vi "CH_LM Measurement Fetch Data.vi"(0 "Meter Index":i32, 3 "All Records? (F)":bool, 5 "error in (no error)":errorcluster, 7 "Timeout / ms (1000)":i32=1000) -> (14 "Meter Index":i32, 16 "Data OK":bool, 17 "Data Array":T1[](array[typedef]) {"Flags" format="%.0b"; "Unit ID" format="%.0b"; "Quad Distance"."Y" format="%#.1f"; "Quad Distance"."X" format="%#.1f"; "Value" format="%#.7e"}, 18 "timed out?":bool, 19 "error out":errorcluster)   [LabVIEW 2017, in "CH_LM.lvlib"]
doc: "This VI reads the streaming data and converts it to LabVIEW datatypes. \nIf the LabMax streaming mode is enabled the streaming data is send with approximatly 10 Hz.\n\n- In case of USB communication mode this VI waits for Streaming Packets.\n- In case of GPIB and RS232 communication mode this VI waits for Service Request (SRQ) and fetches all available data records.\n\n<B>Attention:</B> This VI is intentionally reentrant!\n\n<B>Note:</B> Data without Header is not supported in this revision.\n\nThe meter will internally generate a data record according to the following rules:\n- With every pulse when a pyroelectric probe is attached and if Joules mode is selected\n- Every 300 ms when a pyroelectric probe is attached and if Watts mode is selected\n- With every pulse when a thermopile probe is attached and if Joules mode is selected \n- When a measurement sample is taken when a thermopile or optical probe is attached and if Watts mode is selected\n\nSince thermopile and optical power measurements are continuous in nature (not event based as with pyroelectric probes), the delivery of this data may be configured as a stream of sampled points or simply the last point recorded. Refer to CH_LM Config Measurement Delivery Mode.vi."
uses:
  CH_LM.lvlib
  CH_LM Streaming Data.ctl
  _CH_LM/CH_LM Action Enumeration.ctl
  _CH_LM/CH_LM Event Cluster.ctl
  CH_LM_App/CH_LM Globals Debug-Status.vi
  CH_LM App.lvlib
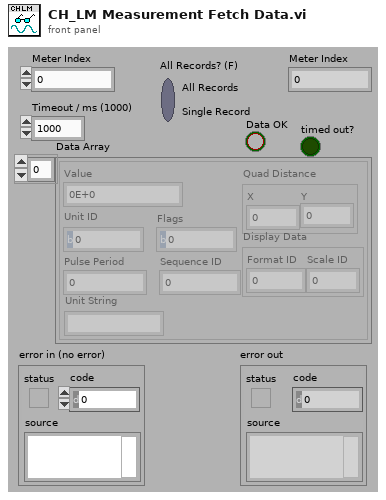
[diagram p1: front panel]
types:
  T1 = typedef "CH_LM.lvlib/CH_LM Streaming Data.ctl" = cluster{"Value":sgl, "Quad Distance":cluster{"X":sgl, "Y":sgl}, "Display Data":cluster{"Format ID":u8, "Scale ID":u8}, "Unit ID":u8, "Flags":u32, "Pulse Period":u32, "Sequence ID":u32, "Unit String":string}
  T2 = typedef "CH_LM.lvlib/CH_LM Action Enumeration.ctl" = enum16{"add", "read", "read by serial", "set", "remove", "delete", "Clear Shift-Register", ""}
  T3 = typedef "CH_LM.lvlib/CH_LM Event Cluster.ctl" = cluster{"Event Name":string, "Meter Index":i32, "Serial  Number":string, "Data":string, "iStreamingPacket":variant}
  T4 = typedef "CH_LM.lvlib/CH_LM Communication Mode.ctl" = enum16{"None", "USB", "GPIB", "RS232"}
  T5 = typedef "CH_LM.lvlib/CH_LM Meter Info.ctl" = cluster{"Meter Index":i32, "Serial Number":string, "Queue Cluster":T6, "Data Header":bool, "Data Tokens":T7[]}
  T6 = typedef "CH_LM.lvlib/CH_LM Queue Cluster.ctl" = cluster{"Streaming Queue":refnum<queue>, "Asynch Notifier":refnum<notifier>}
  T7 = typedef "CH_LM.lvlib/CH_LM Data Token.ctl" = enum16{"Raw data", "Quad distance", "Formated data", "Unit", "Pulse period", "Flags", "Sequence ID"}
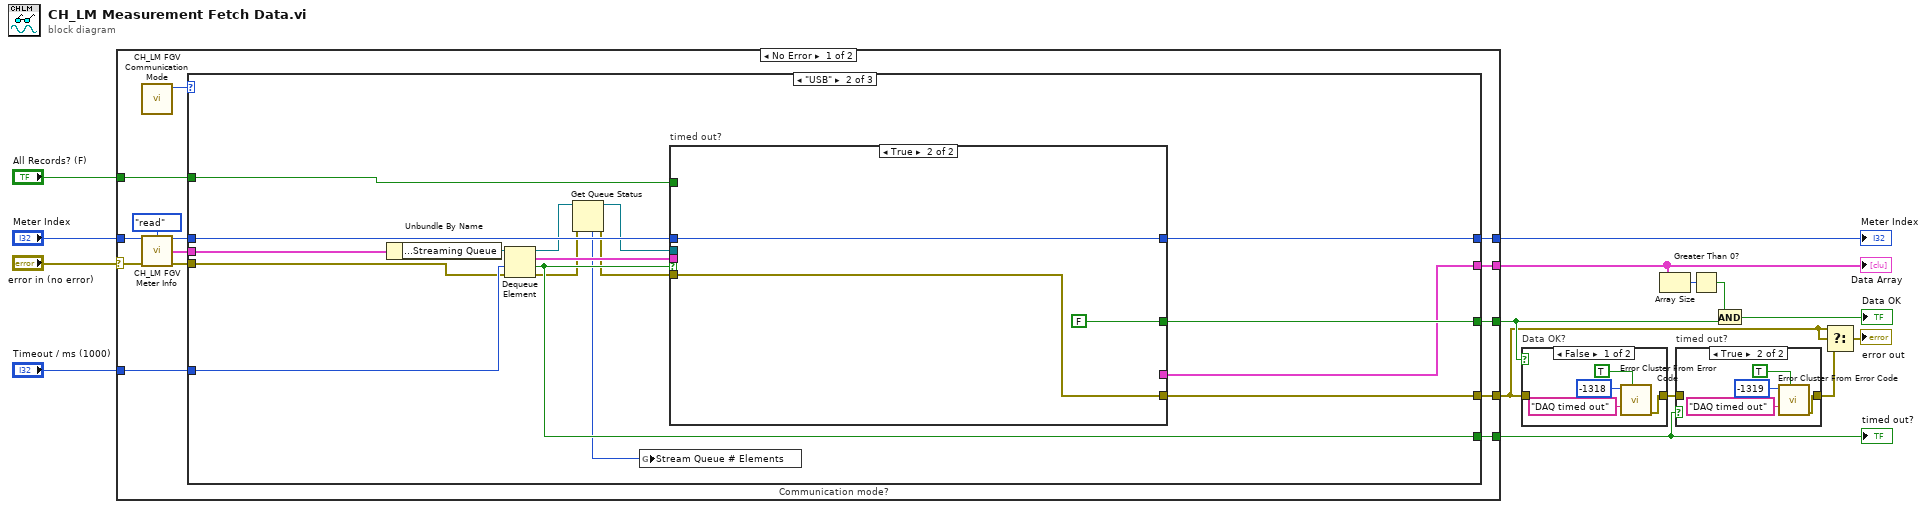
[diagram p0: block diagram]
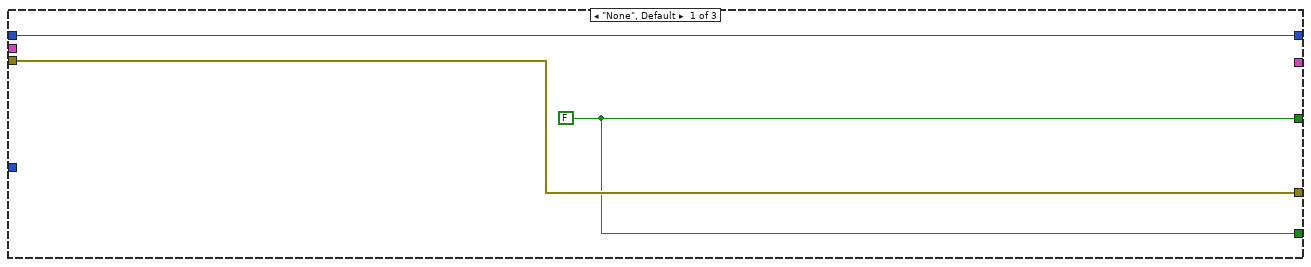
[diagram p4: hidden frame]
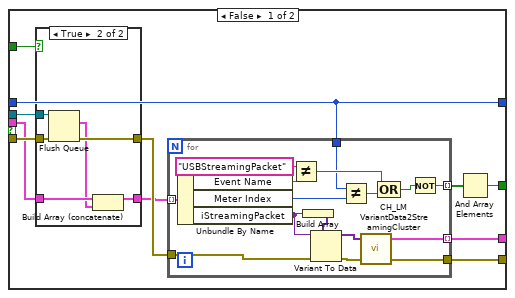
[diagram p5: hidden frame]
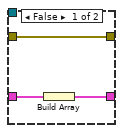
[diagram p6: hidden frame]
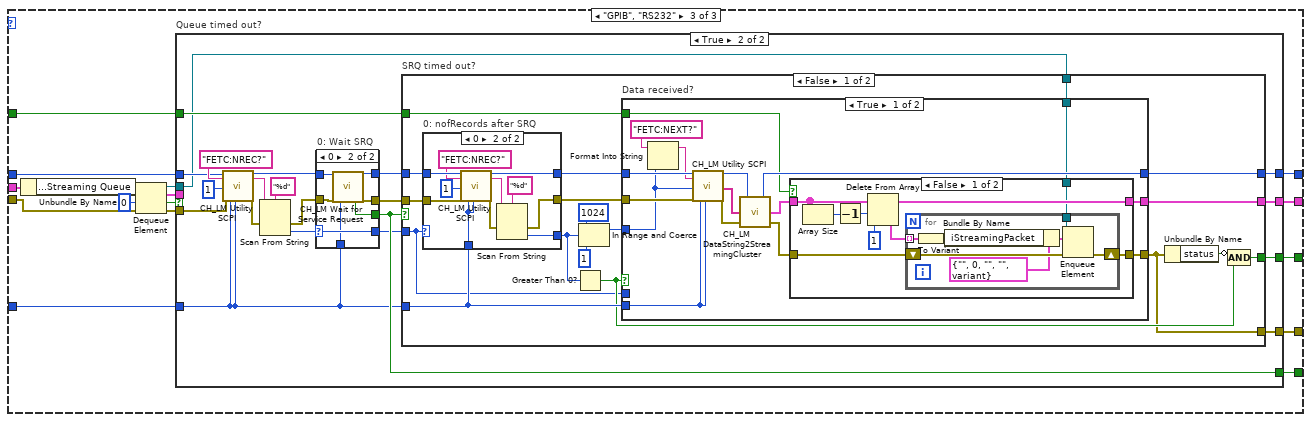
[diagram p7: hidden frame]
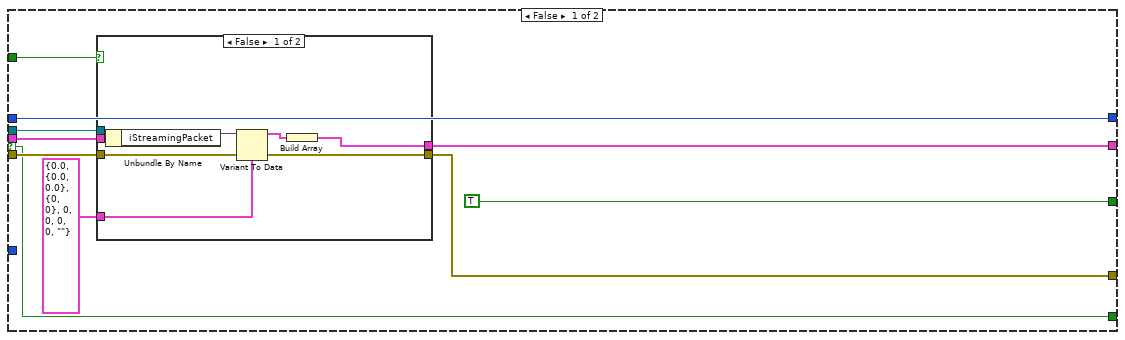
[diagram p8: hidden frame]
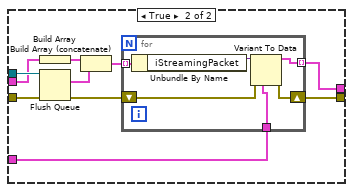
[diagram p9: hidden frame]
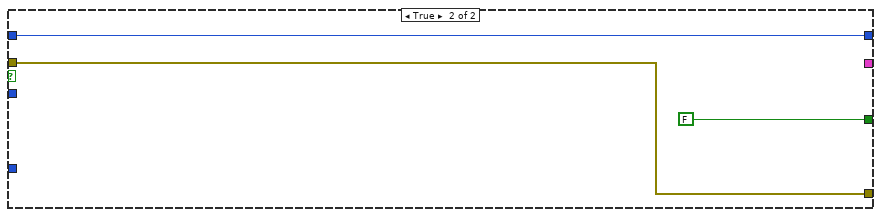
[diagram p14: hidden frame]
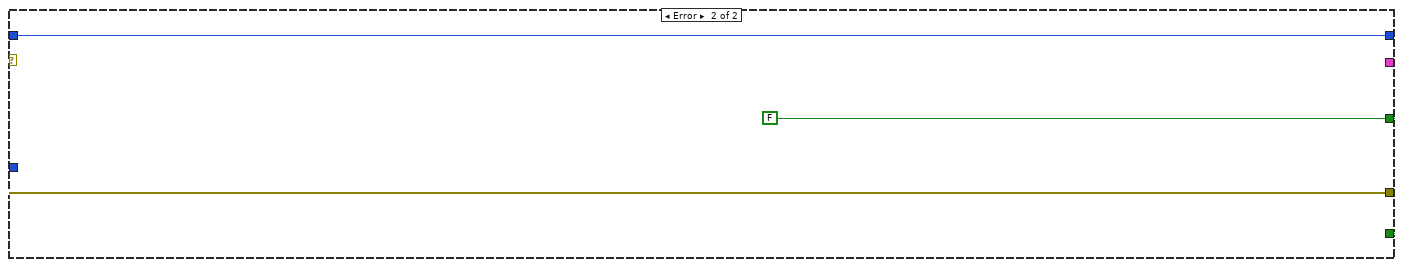
[diagram p15: hidden frame]
diagram:
  n1 = case shown="No Error" "error in (no error)" {
    selector: "error in (no error)" -> [w26 w242]
    tunnel: [w23 w242] -> w3
    tunnel: "Meter Index" -> [w25 w241]
    tunnel: [w19 w241] -> w13
    tunnel: [w22 _] -> w10
    tunnel: [w21 w240] -> w4
    tunnel: "Timeout / ms (1000)" -> [w20 _]
    tunnel: "All Records? (F)" -> [w17 _]
    tunnel: [w16 w240] -> w6
    frame No Error {
      n2 = call "CH_LM FGV Communication Mode.vi"() -> ("Communication Mode"=w18:T4)  [unwired: 3 in, 5 out]
      n3 = call "CH_LM FGV Meter Info.vi"("Meter Index"=w25, "Action (read)"=CH_LM_Action_Enumeration."read", "error in (no error)"=w26) -> ("Meter Index out"=w24:i32, "Meter Info"=w29:T5, "error out"=w28:errorcluster)  [unwired: 2 in, 8 out]
      n4 = case "Communication mode?" shown="\"USB\"" w18 {
        tunnel: w20 -> [_ w49 w97]
        tunnel: w29 -> [_ w48 w96]
        tunnel: w28 -> [w32 w46 w94]
        tunnel: w24 -> [w31 w44 w98]
        tunnel: [w32 w43 w102] -> w23
        tunnel: [_ w38 w103] -> w22
        tunnel: [w30 w45 w101] -> w21
        tunnel: [w31 w42 w104] -> w19
        tunnel: w17 -> [_ w40 w100]
        tunnel: [w30 w39 w99] -> w16
        frame "None", Default {
          w30 = FALSE
        }
        frame "USB" {
          n5 = Unbundle By Name(w48) -> ("Queue Cluster.Streaming Queue"=w47:refnum<queue>)
          n6 = Dequeue Element(queue=w47, timeout in ms (-1)=w49, error in (no error)=w46) -> (queue out=w37:refnum<queue>, element=w41:T3, timed out?=w39:bool, error out=w35:errorcluster)
          n7 = Get Queue Status(queue=w37, error in (no error)=w35) -> (queue out=w36:refnum<queue>, error out=w34:errorcluster, # elements in queue=w33:i32)  [unwired: 1 in, 5 out]
          n8 = global write "CH_LM Globals Debug-Status.vi" "Stream Queue # Elements"(w33) -> ()
          n9 = case "timed out?" shown="True" w39 {
            tunnel: [w59 w86] -> w43
            tunnel: w44 -> [w51 w88]
            tunnel: [w58 _] -> w38
            tunnel: [w57 FALSE] -> w45
            tunnel: w36 -> [w56 _]
            tunnel: w34 -> [w55 w86]
            tunnel: w41 -> [w53 _]
            tunnel: [w51 w88] -> w42
            tunnel: w40 -> [w50 _]
            frame False {
              n10 = case shown="True" w50 {
                tunnel: w56 -> [_ w69]
                tunnel: w55 -> [w63 w68]
                tunnel: [w63 w67] -> w54
                tunnel: w53 -> [w62 w66]
                tunnel: [w61 w64] -> w52
                frame False {
                  n11 = Build Array(w62) -> (w61:T3[])
                }
                frame True {
                  n12 = Flush Queue(queue=w69, error in (no error)=w68) -> (remaining elements=w65:T3[], error out=w67:errorcluster)  [unwired: 1 out]
                  n13 = Build Array (concatenate)(w66, w65) -> (w64:T3[])
                }
              }
              n14 = for {
                tunnel: [w80] -> w60 mode=indexing
                tunnel: [w72] -> w59
                tunnel: w51 -> [w73]
                tunnel: w54 -> [w76]
                tunnel: w52 -> [w75] mode=indexing
                tunnel: [w70] -> w58 mode=indexing
                n15 = Unbundle By Name(w75) -> ("Event Name"=w85:string, "Meter Index"=w77:i32, "iStreamingPacket"=w78:variant)
                n16 = Not Equal?(x="USBStreamingPacket", y=w85) -> (x != y?=w83:bool)
                n17 = Build Array(w78) -> (w79:variant[])
                n18 = Variant To Data(error in=w76, type=w79, Variant=w78) -> (data=w71:variant[], error out=w74:errorcluster)
                n19 = Not Equal?(x=w73, y=w77) -> (x != y?=w82:bool)
                n20 = call "CH_LM VariantData2StreamingCluster.vi"("error in (no error)"=w74, "Streaming Data"=w71) -> ("error out"=w72:errorcluster, "Streaming Data Cluster"=w70:T1)  [unwired: 1 in, 1 out]
                n21 = Compound Arithmetic op=OR(w83, w82) -> (w81:bool)
                n22 = Not(x=w81) -> (.not. x?=w80:bool)
              }
              n23 = And Array Elements(Boolean array=w60) -> (logical AND=w57:bool)
            }
            frame True {
            }
          }
        }
        frame "GPIB", "RS232" {
          n24 = Unbundle By Name(w96) -> ("Queue Cluster.Streaming Queue"=w95:refnum<queue>)
          n25 = Dequeue Element(queue=w95, timeout in ms (-1)=0, error in (no error)=w94) -> (queue out=w89:refnum<queue>, element=w90:T3, timed out?=w91:bool, error out=w93:errorcluster)
          n26 = case "Queue timed out?" shown="True" w91 {
            selector: w91 -> [w107 _]
            tunnel: [w110 w158] -> w104
            tunnel: [w111 w157] -> w103
            tunnel: [w109 w156] -> w102
            tunnel: [TRUE w155] -> w101
            tunnel: w100 -> [w114 w152]
            tunnel: [w107 w151] -> w99
            tunnel: w98 -> [w110 w145]
            tunnel: w97 -> [_ w142]
            tunnel: w93 -> [w112 w139]
            tunnel: w90 -> [w113 _]
            tunnel: w89 -> [w106 w138]
            frame False {
              n27 = case shown="False" w114 {
                tunnel: w113 -> [w121 w130]
                tunnel: w112 -> [w119 w128]
                tunnel: T1 {"Value"=0.0, "Quad Distance"={"X"=0.0, "Y"=0.0}, "Display Data"={"Format ID"=0, "Scale ID"=0}, "Unit ID"=0, "Flags"=0, "Pulse Period"=0, "Sequence ID"=0, "Unit String"=""} ("Streaming Data Cluster") -> [w118 w123]
                tunnel: [w116 w122] -> w111
                tunnel: [w115 w124] -> w109
                tunnel: w106 -> [_ w131]
                frame False {
                  n28 = Unbundle By Name(w121) -> ("iStreamingPacket"=w120:variant)
                  n29 = Variant To Data(error in=w119, type=w118, Variant=w120) -> (data=w117:T1, error out=w115:errorcluster)
                  n30 = Build Array(w117) -> (w116:T1[])
                }
                frame True {
                  n31 = Build Array(w130) -> (w129:T3[])
                  n32 = Flush Queue(queue=w131, error in (no error)=w128) -> (remaining elements=w127:T3[], error out=w125:errorcluster)  [unwired: 1 out]
                  n33 = Build Array (concatenate)(w129, w127) -> (w126:T3[])
                  n34 = for {
                    tunnel: w126 -> [w136] mode=indexing
                    shift-right: [w134] -> w124
                    shift-left: w125 -> [w135]
                    tunnel: w123 -> [w133]
                    tunnel: [w132] -> w122 mode=indexing
                    n35 = Unbundle By Name(w136) -> ("iStreamingPacket"=w137:variant)
                    n36 = Variant To Data(error in=w135, type=w133, Variant=w137) -> (data=w132:T1, error out=w134:errorcluster)
                  }
                }
              }
            }
            frame True {
              n37 = call "CH_LM Utility SCPI.vi"("Meter Index"=w145, "SCPI Command/Query"="FETC:NREC?", "NofStrings (-1:all)"=1, "error in (no error)"=w139, "Timeout / ms (3000)"=w142, "Lock Timeout / ms (1000)"=w142) -> ("Meter Index"=w144:i32, "Response"=w148:string, "error out"=w149:errorcluster)  [unwired: 11 out]
              n38 = Scan From String(format string="%d", input string=w148, error in=w149) -> (error out=w143:errorcluster, output 1=w141:i32)  [unwired: 1 in, 3 out]
              n39 = case "0: Wait SRQ" shown="0" w141 {
                selector: w141 -> [w159 w166]
                tunnel: w144 -> [w161 w168]
                tunnel: [w161 w163] -> w154
                tunnel: w143 -> [w160 w167]
                tunnel: [w160 w162] -> w153
                tunnel: w142 -> [_ w165]
                tunnel: [_ w164] -> w151
                tunnel: [w159 w166] -> w140
                frame Default {
                }
                frame 0 {
                  n40 = call "CH_LM Wait for Service Request.vi"("Meter Index"=w168, "error in (no error)"=w167, "Timeout / ms (1000)"=w165) -> ("timed out?"=w164:bool, "Meter Index"=w163:i32, "error out"=w162:errorcluster)  [unwired: 14 out]
                }
              }
              n41 = case "SRQ timed out?" shown="False" w151 {
                tunnel: [w179 w238] -> w158
                tunnel: [w176 _] -> w157
                tunnel: [w177 w237] -> w156
                tunnel: [w180 FALSE] -> w155
                tunnel: w154 -> [w184 w238]
                tunnel: w153 -> [w183 w237]
                tunnel: w142 -> [w182 _]
                tunnel: w152 -> [w175 _]
                tunnel: w140 -> [w169 _]
                tunnel: w138 -> [w174 _]
                frame False {
                  n42 = case "0: nofRecords after SRQ" shown="0" w169 {
                    selector: w169 -> [w187 _]
                    tunnel: [w189 w200] -> w186
                    tunnel: [w188 w199] -> w185
                    tunnel: w184 -> [w189 w198]
                    tunnel: w183 -> [w188 w197]
                    tunnel: w182 -> [_ w196]
                    tunnel: [w187 w190] -> w173
                    frame Default {
                    }
                    frame 0 {
                      n43 = call "CH_LM Utility SCPI.vi"("Meter Index"=w198, "SCPI Command/Query"="FETC:NREC?", "NofStrings (-1:all)"=1, "error in (no error)"=w197, "Timeout / ms (3000)"=w196, "Lock Timeout / ms (1000)"=w196) -> ("Meter Index"=w200:i32, "Response"=w193:string, "error out"=w192:errorcluster)  [unwired: 11 out]
                      n44 = Scan From String(format string="%d", input string=w193, error in=w192) -> (error out=w199:errorcluster, output 1=w190:i32)  [unwired: 1 in, 3 out]
                    }
                  }
                  n45 = Greater Than 0?(x=w173) -> (x > 0?=w178:bool)
                  n46 = In Range and Coerce(upper limit=1024, x=w173, lower limit=1) -> (coerced(x)=w172:i32)  [unwired: 1 out]
                  n47 = case "Data received?" shown="True" w178 {
                    tunnel: w186 -> [w216 w236]
                    tunnel: w185 -> [w215 w235]
                    tunnel: [w208 w236] -> w179
                    tunnel: [w204 _] -> w176
                    tunnel: [w206 w235] -> w177
                    tunnel: w172 -> [w201 _]
                    tunnel: w182 -> [w213 _]
                    tunnel: w175 -> [w202 _]
                    tunnel: w174 -> [w203 _]
                    tunnel: w169 -> [_ _]
                    frame True {
                      n48 = Format Into String(initial string="FETC:NEXT?" ("SCPI Command/Query"), w201) -> (resulting string=w212:string)  [unwired: 2 in, 1 out]
                      n49 = call "CH_LM Utility SCPI.vi"("Meter Index"=w216, "SCPI Command/Query"=w212, "NofStrings (-1:all)"=w201, "error in (no error)"=w215, "Timeout / ms (3000)"=w213, "Lock Timeout / ms (1000)"=w213) -> ("Meter Index"=w209:i32, "Response Array"=w210:string[], "error out"=w214:errorcluster)  [unwired: 11 out]
                      n50 = call "CH_LM DataString2StreamingCluster.vi"("error in (no error)"=w214, "Data Strings"=w210, "Meter Index"=w209) -> ("error out"=w207:errorcluster, "Data Array"=w205:T1[], "Meter Index out"=w208:i32)
                      n51 = case shown="False" w202 {
                        tunnel: w207 -> [w225 w233]
                        tunnel: [w224 w233] -> w206
                        tunnel: [w222 w234] -> w204
                        tunnel: w205 -> [w219 w234]
                        tunnel: w203 -> [w217 _]
                        frame False {
                          n52 = Array Size(array=w219) -> (size(s)=w220:i32)
                          n53 = Decrement(x=w220) -> (x-1=w218:i32)
                          n54 = Delete From Array(array=w219, length=w218, index=1) -> (deleted portion=w223:T1[], array with subset deleted=w222:T1[])
                          n55 = for {
                            tunnel: w223 -> [w230] mode=indexing
                            tunnel: w217 -> [w229]
                            shift-right: [w231] -> w224
                            shift-left: w225 -> [w232]
                            n56 = To Variant(anything=w230) -> (Variant=w226:variant)
                            n57 = Bundle By Name(cluster=T3 {"Event Name"="", "Meter Index"=0, "Serial  Number"="", "Data"="", "iStreamingPacket"=variant} ("element"), "iStreamingPacket"=w226) -> (w228:T3)
                            n58 = Enqueue Element(queue=w229, element=w228, error in (no error)=w232) -> (error out=w231:errorcluster)  [unwired: 3 out]
                          }
                        }
                        frame True {
                        }
                      }
                    }
                    frame False {
                    }
                  }
                  n59 = Unbundle By Name(w177) -> ("status"=w181:bool)
                  n60 = Compound Arithmetic op=AND(invert w181, w178) -> (w180:bool)
                }
                frame True {
                }
              }
            }
          }
        }
      }
    }
    frame Error {
      w240 = FALSE
    }
  }
  "Meter Index" <- w13
  "Data Array" <- w10
  "timed out?" <- w6
  n61 = case "Data OK?" shown="False" w4 {
    tunnel: [w244 w247] -> w5
    tunnel: w3 -> [_ w247]
    frame False {
      n62 = call <vilib>:"Error Cluster From Error Code.vi"("show call chain? (False)"=TRUE, "error message (\"\")"="DAQ timed out" ("error message (\"\")"), "error code (0)"=-1318) -> ("error out"=w244:errorcluster)  [unwired: 1 in, 5 out]
    }
    frame True {
    }
  }
  n63 = Array Size(array=w10) -> (size(s)=w9:i32)
  n64 = case "timed out?" shown="True" w6 {
    tunnel: [w248 w250] -> w1
    tunnel: w5 -> [w248 _]
    frame False {
    }
    frame True {
      n65 = call <vilib>:"Error Cluster From Error Code.vi"("show call chain? (False)"=TRUE, "error message (\"\")"="DAQ timed out" ("error message (\"\")"), "error code (0)"=-1319) -> ("error out"=w250:errorcluster)  [unwired: 1 in, 5 out]
    }
  }
  n66 = Greater Than 0?(x=w9) -> (x > 0?=w8:bool)
  n67 = And(x=w8, y=w4) -> (x .and. y?=→"Data OK":bool)
  n68 = Select(t=w3, s=w3, f=w1) -> (s? t:f=→"error out":errorcluster)
